vi "Mono_initJPJ.vi"(8 "error in (no error)":errorcluster) -> (0 "error out":errorcluster, 1 "Mono Connected?":bool, 3 "CmdLib":refnum<k24>)   [LabVIEW 2017]
uses:
  C:/Users/Admin/Desktop/Sensitive EQE Stuff/S-EQE (YJ)/Mono vi (YJ)/Cornerstone.dll
  Cornerstone.dll
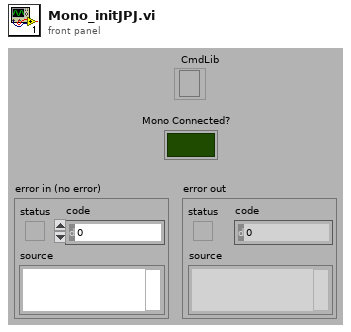
[diagram p1: front panel]
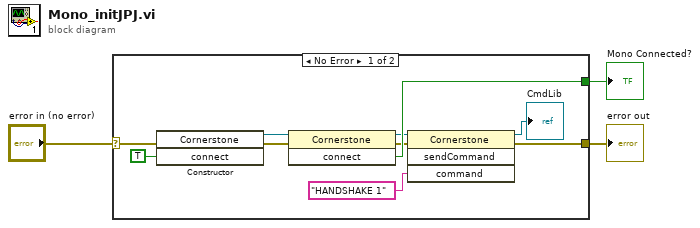
[diagram p0: block diagram]
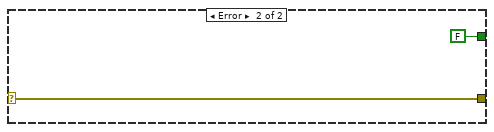
[diagram p2: hidden frame]
diagram:
  n1 = case shown="No Error" "error in (no error)" {
    selector: "error in (no error)" -> [w13 w15]
    tunnel: [w4 w15] -> w2
    tunnel: [w9 FALSE] -> w1
    frame No Error {
      n2 = constructor class="Cornerstone"(error in=w13, "connect"=TRUE) -> (reference out=w11:refnum<k24>, error out=w10:errorcluster)  [unwired: 2 in, 2 out]
      n3 = invoke class="Cornerstone" method="connect"(reference=w11, error in=w10) -> (reference out=w8:refnum<k24>, error out=w5:errorcluster, "connect"=w9:bool)  [unwired: 1 in]
      n4 = invoke class="Cornerstone" method="sendCommand"(reference=w8, error in=w5, "command"="HANDSHAKE 1") -> (reference out=→"CmdLib":refnum<k24>, error out=w4:errorcluster)  [unwired: 1 in, 2 out]
    }
    frame Error {
    }
  }
  "error out" <- w2
  "Mono Connected?" <- w1
